vi "FlatToRichcif_channelcore_Channels.vi"(5 "OutputClusterType":T1, 11 "InputCluster":T5) -> (3 "OutputCluster":T1)   [LabVIEW 2021, in "CIF_PluginLoader_server.lvlib"]
uses:
  CIF_PluginLoader_server.lvlib
  cif_channelcore_Channels_Flat.ctl
  cif_channelcore_Channel_Flat.ctl
  cif_channelcore_ChannelDirection.ctl
  cif_channelcore_ChannelPattern.ctl
  cif_channelcore_Channels.ctl
  cif_channelcore_Channel.ctl
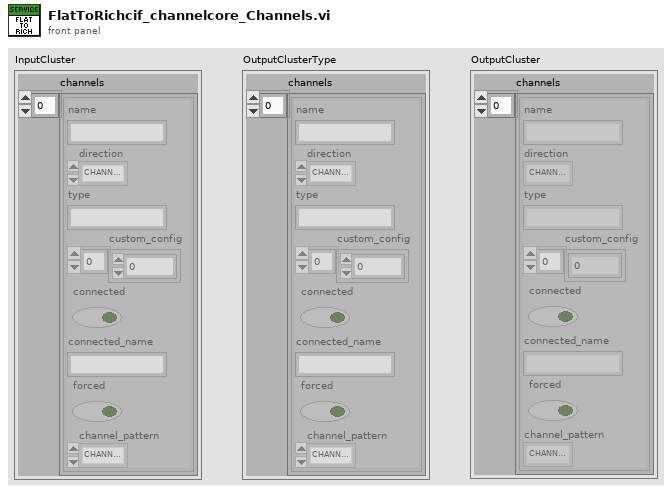
[diagram p1: front panel]
types:
  T1 = typedef "CIF_PluginLoader_server.lvlib/cif_channelcore_Channels.ctl" = cluster{"channels":T2[]}
  T2 = typedef "CIF_PluginLoader_server.lvlib/cif_channelcore_Channel.ctl" = cluster{"name":string, "direction":T3, "type":string, "custom_config":u8[], "connected":bool, "connected_name":string, "forced":bool, "channel_pattern":T4}
  T3 = typedef "CIF_PluginLoader_server.lvlib/cif_channelcore_ChannelDirection.ctl" = enum32{"CHANNELDIRECTION_UNKNOWN", "CHANNELDIRECTION_PUBLISHER", "CHANNELDIRECTION_SUBSCRIBER"}
  T4 = typedef "CIF_PluginLoader_server.lvlib/cif_channelcore_ChannelPattern.ctl" = enum32{"CHANNELPATTERN_UNKNOWN", "CHANNELPATTERN_TAG", "CHANNELPATTERN_FIFO", "CHANNELPATTERN_MULTIFIFO", "CHANNELPATTERN_BACKPRESSUREFIFO"}
  T5 = typedef "CIF_PluginLoader_server.lvlib/cif_channelcore_Channels_Flat.ctl" = cluster{"channels":T6[]}
  T6 = typedef "CIF_PluginLoader_server.lvlib/cif_channelcore_Channel_Flat.ctl" = cluster{"name":string, "direction":T3, "type":string, "custom_config":u8[], "connected":bool, "connected_name":string, "forced":bool, "channel_pattern":T4}
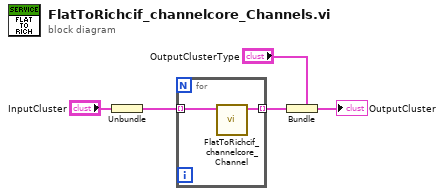
[diagram p0: block diagram]
diagram:
  n1 = Unbundle "Unbundle"("InputCluster") -> ("channels"=w2:T6[])
  n2 = for {
    tunnel: w2 -> [w7] mode=indexing
    tunnel: [w6] -> w1 mode=indexing
    n3 = call "FlatToRichcif_channelcore_Channel.vi"("InputCluster"=w7) -> ("OutputCluster"=w6:T2)  [unwired: 10 in]
  }
  n4 = Bundle "Bundle"(cluster="OutputClusterType", "channels"=w1) -> (→"OutputCluster":T1)
